vi "PWM Servo FPGA.vi"(8 "Disable\nDrive":bool, 9 "Enable\nDrive":bool, 10 "Position Setpoint":i32 caption="Setpoint") -> (0 "Trig AI":bool, 3 "Encoder Position":i32)   [LabVIEW 2012]
doc: "This VI shows an example of how to implement a closed loop position move using the NI 9505. The position loop is implemented using PID. The output of the loop is used as the command for the current loop, which then sets the PWM duty cycle for the motor. This example assumes that an encoder is connected for position and velocity feedback. This example does not implement advanced motion features such as trajectory generation and splining."
uses:
  <vilib>/LabVIEW Targets/FPGA/cRIO/cRIO-9505/controls.llb/_nicrio_cRIO-9505_DriveStatus.ctl
  <vilib>/Platform/TimedLoop/XDataNode/timing_clust.ctl
  <vilib>/Platform/TimedLoop/XDataNode/nitl_modes.ctl
  <vilib>/Platform/TimedLoop/XDataNode/wakeup.ctl
  <vilib>/LabVIEW Targets/FPGA/cRIO/cRIO-9505/controls.llb/_nicrio_cRIO-9505_DriveDirection.ctl
  Instance           1 55Saved   Position Control (closed loop) - NI 9505 (FPGA) .vi
  <vilib>/rvi/Emulation/niFpgaSctlEmulationRegisterWithScheduler.vi
  <vilib>/rvi/Emulation/niFpgaSctlEmulationScheduler.vi
  <vilib>/rvi/eio/common/nirviEmuTemplateMethod_errors.vi
  Instance           2 55Saved   Position Control (closed loop) - NI 9505 (FPGA) .vi
  Instance           3 55Saved   Position Control (closed loop) - NI 9505 (FPGA) .vi
  <vilib>/rvi/eio/common/nirviEmuTemplatePropertyGet_noerrors.vi
  Instance           4 55Saved   Position Control (closed loop) - NI 9505 (FPGA) .vi
  <vilib>/Platform/TimedLoop/XDataNode/XDataNode.xnode
  <vilib>/eio/EIONode/EIONode.xnode
  <vilib>/addons/control/pid/fpga.llb/XNode/niFpgaPID.xnode
  <vilib>/eio/EIOMethodNode/EIOMethodNode.xnode
  <vilib>/eio/EIOPropertyNode/EIOPropertyNode.xnode
  <vilib>/Platform/TimedLoop/XDataNode/XDNodeRunTimeDep.lvlib
  <vilib>/rvi/eio/common/nirviEmuTemplatePropertyGet_errors.vi
  <vilib>/rvi/eio/common/nirviEmuTemplatePropertySet_errors.vi
  <vilib>/rvi/eio/common/nirviEmuTemplatePropertySet_noerrors.vi
panel:
  out "Current Feedback":i16
  in  "PID gains":T1={"proportional gain (Kc)"=20.0, "integral gain (Kc*Ts/Ti)"=10.0, "derivative gain (Kc*Td/Ts)"=0.0}
  in  "Current Limit":i16=806
  in  "Current Loop Rate (usec)":u16=50
  in  "Position PID Gains":T2={"Kp"=50, "Kd"=1000, "Ki"=0, "ILim"=1000, "Kv"=0, "Vff"=0, "Aff"=0, "Td"=0}
  out "Vsup Present":bool
  out "Drive Fault":bool
  out "Drive Status":T3=enum."Disabled"
  out "Temp Fault":bool
  in  "Position Loop  Rate (usec)":u16=250
  in  "Position Error Limit":i16=32767
  out "Position Error Read":i16
  out "Position Error Status":bool
  out "Current Loop Output":i16
  out "Current Command":i16
  in  "Reset Position":bool
  in  "Reset Position Value":i32
  out "ticks/count":u32
  out "Index (Z) Position":i32
  out "counts (no reset)":i32
  # "These parameters control the response of the position loop. Position Setpoint is the desired position to go to. Position Error Limit is the maximum allowed error the setpoint and actual position returned by the encoder loop."
  # "These parameters control the response\nof the current loop. The current limit is the \nmaximum current allowed."
  # "Use \"Enable Drive\" and \"Disable Drive\" to \nturn start and stop motor"
  # "Current Loop Parameters"
  # "Enter Position Setpoint\nto manually move the\nmotor"
  # "These status controls/indicators are used to enable/disable the drive and read fault information."
  # "Use the Reset Position control to reset the quadrature count to the value in Reset Position Value."
  # "Drive Status"
  # "Position Loop Parameters"
  # "Encoder Parameters"
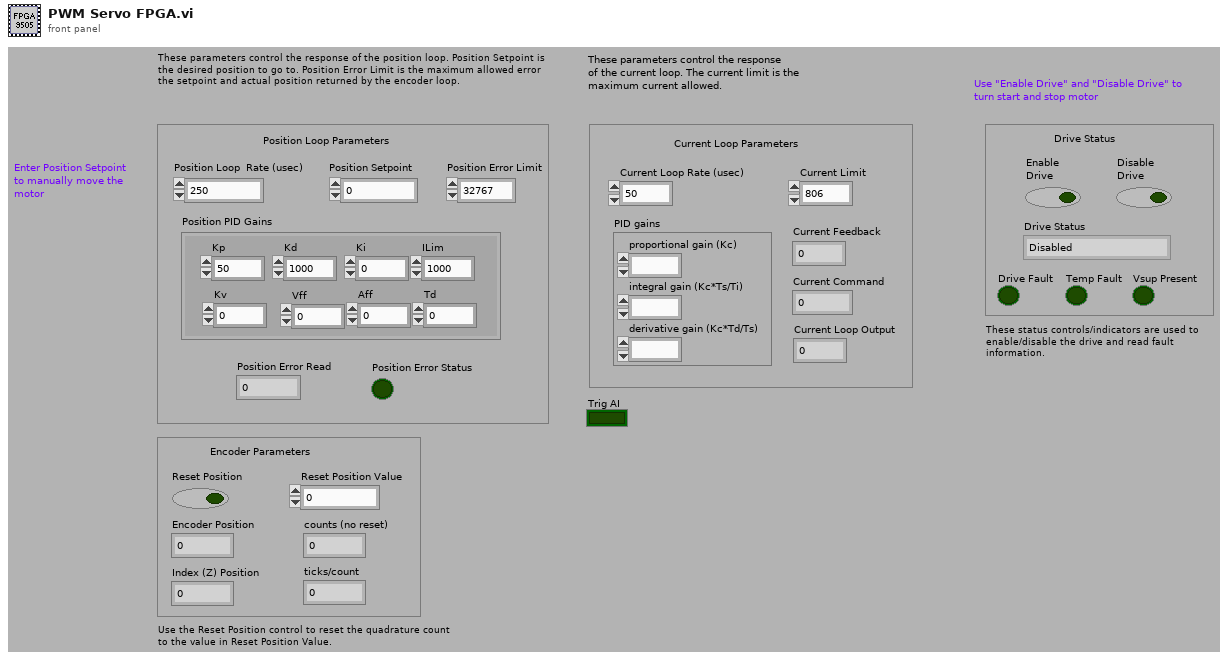
[diagram p1: front panel]
types:
  T1 = cluster{"proportional gain (Kc)":fxp<+/-,16,8>, "integral gain (Kc*Ts/Ti)":fxp<+/-,16,8>, "derivative gain (Kc*Td/Ts)":fxp<+/-,16,8>}
  T2 = cluster{"Kp":i16, "Kd":i16, "Ki":i16, "ILim":i16, "Kv":i16, "Vff":i16, "Aff":i16, "Td":i16}
  T3 = typedef "_nicrio_cRIO-9505_DriveStatus.ctl" = enum8{"Enabled", "Disabled", "Disabled by Drive Fault", "Disabled by Temp. Fault", "Disabled by E-Stop", "Unknown"}
  T4 = typedef "XDNodeRunTimeDep.lvlib/timing_clust.ctl" = cluster{"Expected End [f-1]":u64, "Actual End [f-1]":u64, "Finished Late? [f-1]":bool, "Expected End [i-1]":u64, "Actual End [i-1]":u64, "Finished Late? [i-1]":bool, "Expected Start [i]":u64, "Actual Start [i]":u64, "Expected Start [f]":u64, "Actual Start [f]":u64, "Source Name":string, "Structure Name":string, "Period":i64, "Deadline":i64, "Offset":i64, "Start":i64, "Priority":i32, "Timeout":i32, "Mode":T5, "Wakeup Reason":T6, "Error":errorcluster, "Source Type":string, "Secondary Source Type":string, "Global End Time":u64, "Global Start Time":u64, "Frame Duration":u64, "Iteration Duration":u64, "Assigned CPU":i32, "I/O Scan Engine Mode":u32}
  T5 = typedef "XDNodeRunTimeDep.lvlib/nitl_modes.ctl" = enum32{"No Change", "Process missed periods, maintain original phase", "Discard missed periods, maintain original phase", "Process missed periods, ignore original phase", "Discard missed periods, ignore original phase"}
  T6 = typedef "XDNodeRunTimeDep.lvlib/wakeup.ctl" = enum32{"Normal", "Aborted", "Asynchronous wakeup", "Timing source error", "Timed loop error", "Timeout"}
  T7 = cluster{"proportional gain (Kc)":i16, "integral gain (Kc*Ts/Ti)":i16, "derivative gain (Kc*Td/Ts)":i16}
  T8 = typedef "_nicrio_cRIO-9505_DriveDirection.ctl" = enum8{"Clockwise", "Counterclockwise"}
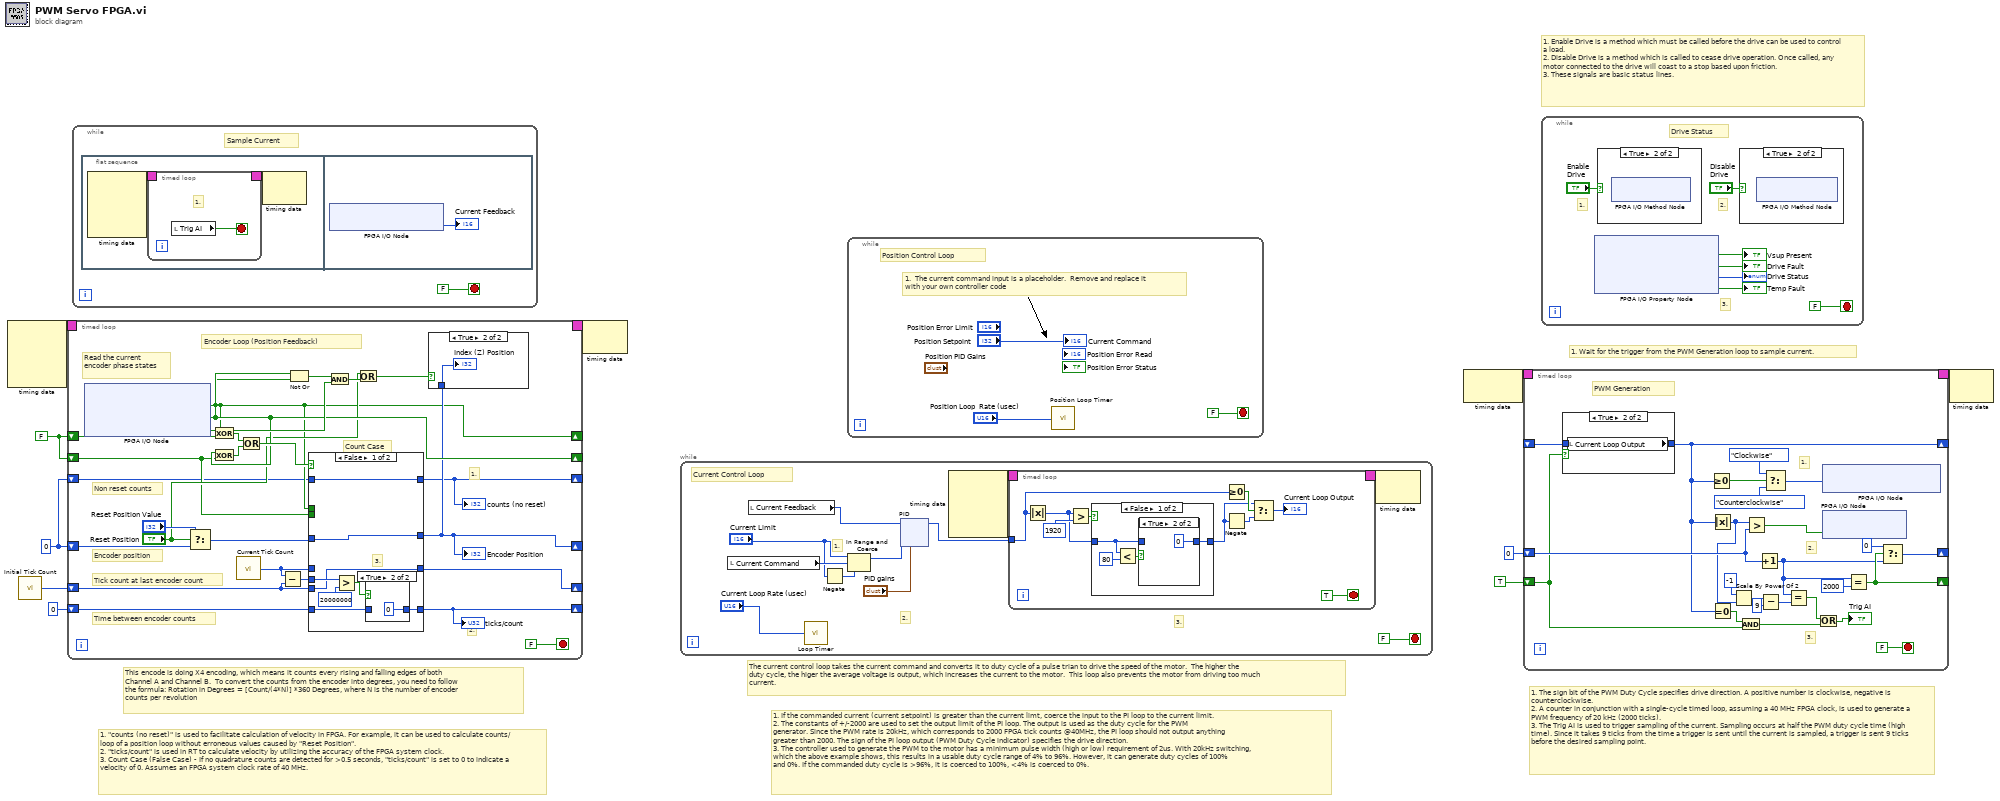
[diagram p0: block diagram]
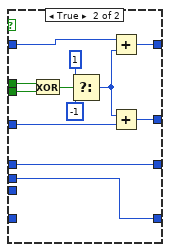
[diagram p4: hidden frame]
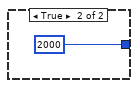
[diagram p7: hidden frame]
diagram:
  w1 = 0 ("Reset Position Value")
  w4 = FALSE ("Encoder Phase A")
  # "The current control loop takes the current command and converts it to duty cycle of a pulse trian to drive the speed of the motor.  The higher the\nduty cycle, the higer the average voltage is output, which increases the current to the motor.  This loop also prevents the motor from driving too much \ncurrent."
  # "This encode is doing X4 encoding, which means it counts every rising and falling edges of both\nChannel A and Channel B.  To convert the counts from the encoder into degrees, you need to follow \nthe formula: Rotation in Degrees = [Count/(4*N)] *360 Degrees, where N is the number of encoder\ncounts per revolution"
  # "1. \"counts (no reset)\" is used to facilitate calculation of velocity in FPGA. For example, it can be used to calculate counts/loop of a position loop without erroneous values caused by \"Reset Position\". \n2. \"ticks/count\" is used in RT to calculate velocity by utilizing the accuracy of the FPGA system clock.\n3. Count Case (False Case) - If no quadrature counts are detected for >0.5 seconds, \"ticks/count\" is set to 0 to indicate a velocity of 0. Assumes an FPGA system clock rate of 40 MHz."
  # "1. Enable Drive is a method which must be called before the drive can be used to control a load.\n2. Disable Drive is a method which is called to cease drive operation. Once called, any motor connected to the drive will coast to a stop based upon friction.\n3. These signals are basic status lines."
  # "1. The sign bit of the PWM Duty Cycle specifies drive direction. A positive number is clockwise, negative is counterclockwise. \n2. A counter in conjunction with a single-cycle timed loop, assuming a 40 MHz FPGA clock, is used to generate a PWM frequency of 20 kHz (2000 ticks).\n3. The Trig AI is used to trigger sampling of the current. Sampling occurs at half the PWM duty cycle time (high time). Since it takes 9 ticks from the time a trigger is sent until the current is sampled, a trigger is sent 9 ticks before the desired sampling point."
  # "1. Wait for the trigger from the PWM Generation loop to sample current."
  # "1. If the commanded current (current setpoint) is greater than the current limt, coerce the input to the PI loop to the current limit.\n2. The constants of +/-2000 are used to set the output limit of the PI loop. The output is used as the duty cycle for the PWM\ngenerator. Since the PWM rate is 20kHz, which corresponds to 2000 FPGA tick counts @40MHz, the PI loop should not output anything\ngreater than 2000. The sign of the PI loop output (PWM Duty Cycle indicator) specifies the drive direction.\n3. The controller used to generate the PWM to the motor has a minimum pulse width (high or low) requirement of 2us. With 20kHz switching,\nwhich the above example shows, this results in a usable duty cycle range of 4% to 96%. However, it can generate duty cycles of 100%\nand 0%. If the commanded duty cycle is >96%, it is coerced to 100%, <4% is coerced to 0%."
  n1 = node-c288() -> (w6:T4)  [unwired: 4 out]
  n2 = call "Initial Tick Count"() -> ("Tick Count(Ticks)"=w3:u32)
  n3 = timed-loop {
    shift-right: [w17] -> _
    shift-left: w4 -> [w35]
    shift-right: [w23] -> _
    shift-left: w4 -> [w16]
    shift-right: [w19] -> _
    shift-left: w1 -> [w32]
    shift-right: [w28] -> _
    shift-left: w3 -> [w12]
    shift-right: [w27] -> _
    shift-left: u32 0 -> [w26]
    timing: w6 -> [_]
    timing-out: [_] -> w5
    shift-right: [w14] -> _
    shift-left: w1 -> [w15]
    stop <- FALSE stop-if-true
    # "Count Case"
    # "Encoder Loop (Position Feedback)"
    # "2."
    # "1."
    # "Read the current\nencoder phase states"
    # "Non reset counts"
    # "Encoder position"
    # "Time between encoder counts"
    # "Tick count at last encoder count"
    n4 = xnode "FPGA I/O Node"() -> ("Mod7/Encoder Phase A"=w17:bool, "Mod7/Encoder Phase B"=w23:bool, "Mod7/Encoder Index"=w24:bool)  [unwired: 3 in, 3 out]
    n5 = Select(t="Reset Position Value", s="Reset Position", f=w32) -> (s? t:f=w30:i32)
    n6 = Exclusive Or(1:w35, 2:w17) -> (0:w34:bool)
    n7 = Exclusive Or(1:w16, 2:w23) -> (0:w33:bool)
    n8 = call "Current Tick Count"() -> ("Tick Count(Ticks)"=w13:u32)
    n9 = Or(x=w34, y=w33) -> (x .or. y?=w31:bool)
    n10 = Subtract(x=w13, y=w12) -> (x-y=w11:u32)
    n11 = Not Or(1:w17, 2:w23) -> (0:w21:bool)
    n12 = case shown="False" w31 {
      tunnel: [w44 w52] -> w19
      tunnel: w30 -> [w44 w58]
      tunnel: w13 -> [_ w48]
      tunnel: [w39 w48] -> w28
      tunnel: w12 -> [w39 _]
      tunnel: [w37 w47] -> w27
      tunnel: w26 -> [w38 _]
      tunnel: w17 -> [_ w54]
      tunnel: w16 -> [_ w53]
      tunnel: [w43 w50] -> w14
      tunnel: w15 -> [w43 w49]
      tunnel: w11 -> [w40 w47]
      frame False {
        # "3."
        n13 = Greater?(x=w40, y=20000000 ("x")) -> (0:w41:bool)
        n14 = case shown="True" w41 {
          tunnel: [w45 u32 0] -> w37
          tunnel: w38 -> [w45 _]
          frame False {
          }
          frame True {
          }
        }
      }
      frame True {
        n15 = Exclusive Or(1:w53, 2:w54) -> (0:w55:bool)
        n16 = Select(t=1 ("16 bit"), s=w55, f=-1 ("16 bit")) -> (s? t:f=w51:i32)
        n17 = Add(x=w49, y=w51) -> (x+y=w50:i32)
        n18 = Add(x=w51, y=w58) -> (x+y=w52:i32)
      }
    }
    "Encoder Position" <- w19
    "ticks/count" <- w27
    "counts (no reset)" <- w14
    n19 = And(x=w21, y=w24) -> (x .and. y?=w22:bool)
    n20 = Or(x="Reset Position", y=w22) -> (x .or. y?=w20:bool)
    n21 = case shown="True" w20 {
      tunnel: w19 -> [_ w36]
      frame False {
      }
      frame True {
        "Index (Z) Position" <- w36
      }
    }
  }
  n22 = while {
    stop <- FALSE stop-if-true
    # "Sample Current"
    n23 = flat-sequence {
      frame #0 {
        n24 = node-c288() -> (w63:T4)  [unwired: 4 out]
        n25 = timed-loop {
          timing: w63 -> [_]
          timing-out: [_] -> w62
          stop <- w64 stop-if-true
          # "1."
          n26 = local read "Trig AI"() -> (w64:bool)
        }
        n27 = node-c288(w62) -> ()  [unwired: 1 out]
      }
      frame #1 {
        n28 = xnode "FPGA I/O Node"() -> ("Mod7/Current Sense"=→"Current Feedback":i16)  [unwired: 1 in, 1 out]
      }
    }
  }
  n29 = node-c288(w5) -> ()  [unwired: 1 out]
  n30 = while {
    stop <- FALSE stop-if-true
    # "3."
    # "2."
    # "1."
    # "Current Control Loop"
    n31 = local read "Current Command"() -> (w76:i16)
    n32 = local read "Current Feedback"() -> (w70:i16)
    n33 = call "Loop Timer"("Count(uSec)"="Current Loop Rate (usec)") -> ()  [unwired: 1 out]
    n34 = Negate(x="Current Limit") -> (-x=w77:i16)
    n35 = In Range and Coerce(upper limit="Current Limit", x=w76, lower limit=w77) -> (coerced(x)=w73:i16)  [unwired: 1 out]
    n36 = xnode "PID"("process variable"=w70, "setpoint"=w73, "PID gains"="PID gains") -> ("output"=w71:i16)  [unwired: 2 in]
    n37 = node-c288() -> (w79:T4)  [unwired: 4 out]
    n38 = timed-loop {
      timing: w79 -> [_]
      timing-out: [_] -> w78
      tunnel: w71 -> [w111]
      stop <- TRUE stop-if-true
      n39 = Absolute Value(x=w111) -> (abs(x)=w112:i16)
      n40 = Greater?(x=w112, y=i16 1920 ("upper limit")) -> (0:w114:bool)
      n41 = case shown="False" w114 {
        tunnel: [w120 i16 2000 ("upper limit")] -> w113
        tunnel: w112 -> [w118 _]
        frame False {
          n42 = Less?(x=w118, y=i16 80 ("lower limit")) -> (x < y?=w119:bool)
          n43 = case shown="True" w119 {
            tunnel: [w122 i16 0 ("upper limit")] -> w120
            tunnel: w118 -> [w122 _]
            frame False {
            }
            frame True {
            }
          }
        }
        frame True {
        }
      }
      n44 = Greater Or Equal To 0?(x=w111) -> (x >= 0?=w117:bool)
      n45 = Negate(x=w113) -> (-x=w116:i16)
      n46 = Select(t=w113, s=w117, f=w116) -> (s? t:f=→"Current Loop Output":i16)
    }
    n47 = node-c288(w78) -> ()  [unwired: 1 out]
  }
  n48 = while "Position Control Loop" {
    stop <- FALSE stop-if-true
    # "1.  The current command input is a placeholder.  Remove and replace it\nwith your own controller code"
    # "Position Control Loop"
    n49 = call "Position Loop Timer"("Count(uSec)"="Position Loop  Rate (usec)") -> ()  [unwired: 1 out]
    "Current Command" <- "Position Setpoint"
  }
  n50 = node-c288() -> (w10:T4)  [unwired: 1 out]
  n51 = timed-loop {
    timing: w10 -> [_]
    timing-out: [_] -> w9
    shift-right: [w152] -> _
    shift-left: i16 0 -> [w155]
    shift-right: [w151] -> _
    shift-left: TRUE -> [w148]
    shift-right: [w135] -> _
    shift-left: _ -> [w150]
    stop <- FALSE stop-if-true
    # "3."
    # "2."
    # "1."
    # "PWM Generation"
    n52 = case shown="True" w148 {
      tunnel: [w156 w157] -> w135
      tunnel: w150 -> [w156 _]
      frame False {
      }
      frame True {
        n53 = local read "Current Loop Output"() -> (w157:i16)
      }
    }
    n54 = Greater Or Equal To 0?(x=w135) -> (x >= 0?=w144:bool)
    n55 = Absolute Value(x=w135) -> (abs(x)=w133:i16)
    n56 = Equal To 0?(x=w135) -> (x = 0?=w149:bool)
    n57 = Scale By Power Of 2(n=i8 -1, x=w133) -> (x*2^n=w137:i16)
    n58 = And(x=w149, y=w148) -> (x .and. y?=w145:bool)
    n59 = Greater?(x=w133, y=w155) -> (0:w141:bool)
    n60 = Increment(x=w155) -> (x+1=w147:i16)
    n61 = Subtract(x=w137, y=i8 9) -> (x-y=w136:i16)
    n62 = Select(t=_nicrio_cRIO-9505_DriveDirection."Clockwise" ("Drive Direction"), s=w144, f=_nicrio_cRIO-9505_DriveDirection."Counterclockwise" ("Drive Direction")) -> (s? t:f=w140:T8)
    n63 = Equal?(x=w147, y=w136) -> (x = y?=w146:bool)
    n64 = Or(x=w146, y=w145) -> (x .or. y?=→"Trig AI":bool)
    n65 = xnode "FPGA I/O Node"("Mod7/Drive Direction"=w140) -> ()  [unwired: 1 in, 1 out]
    n66 = xnode "FPGA I/O Node"("Mod7/Motor"=w141) -> ()  [unwired: 1 in, 1 out]
    n67 = Equal?(x=w147, y=i16 2000) -> (x = y?=w151:bool)
    n68 = Select(t=i16 0, s=w151, f=w147) -> (s? t:f=w152:i16)
  }
  n69 = while {
    stop <- FALSE stop-if-true
    # "Drive Status"
    # "3."
    # "2."
    # "1."
    n70 = xnode "FPGA I/O Property Node"() -> ("Vsup Present"=→"Vsup Present":bool, "Drive Fault"=→"Drive Fault":bool, "Drive Status"=→"Drive Status":T3, "Over Temperature Fault"=→"Temp Fault":bool)  [unwired: 1 in, 1 out]
    n71 = case shown="True" "Enable\nDrive" {
      frame False {
      }
      frame True {
        n72 = xnode "FPGA I/O Method Node"() -> ()  [unwired: 1 in, 1 out]
      }
    }
    n73 = case shown="True" "Disable\nDrive" {
      frame False {
      }
      frame True {
        n74 = xnode "FPGA I/O Method Node"() -> ()  [unwired: 1 in, 1 out]
      }
    }
  }
  n75 = node-c288(w9) -> ()  [unwired: 1 out]
